vi "Number to Match.vi"() -> ()   [LabVIEW 2024]
uses:
  <vilib>/numeric/Random Number (Range) U64.vi
  <vilib>/numeric/sub_Random U32.vi
panel:
  in  "Stop":bool
  out "Iteration count":i32
  in  "Number to match":dbl
  # "Guidance\n1. Click on the numeric control \"Number to match\" and set its value as an integer between 0 and 100. (If you input an integer beyond the range or a noninteger, the program will never stop automatically, so please click the \"STOP\" button to stop the program manually)\n2. Run the application.\n3. The numeric indicator \"Iteration count\" will show the number of iterations the embedded random number generator takes to match the given integer."
  # "Input"
  # "Output"
  # "An integer between 0 and 100"
  # "An integer beyond the range or a noninteger"
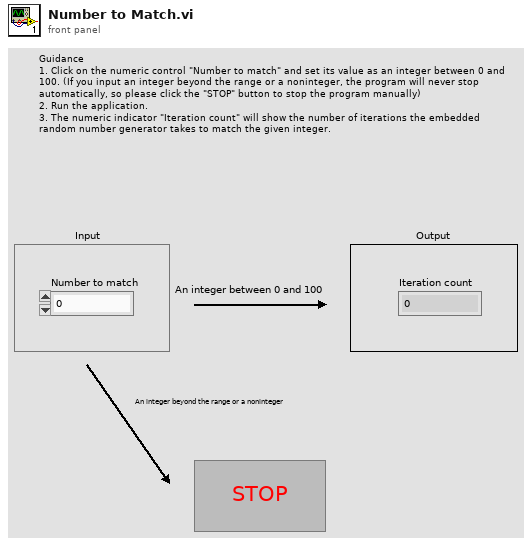
[diagram p1: front panel]
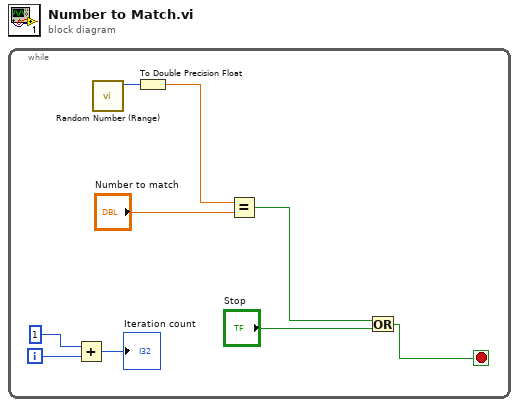
[diagram p0: block diagram]
diagram:
  n1 = while {
    i -> [w6]
    stop <- w1 stop-if-true
    n2 = Add(x=1, y=w6) -> (x+y=→"Iteration count":i32)
    n3 = call-poly <vilib>:"Random Number (Range).vi"() -> ("number"=w8:u64)  [unwired: 11 in]
    n4 = To Double Precision Float(number=w8) -> (double precision float=w7:dbl)
    n5 = Equal?(x=w7, y="Number to match") -> (x = y?=w2:bool)
    n6 = Or(x=w2, y="Stop") -> (x .or. y?=w1:bool)
  }
